vi "MainVI.vi"() -> ()   [LabVIEW 2013]
uses:
  Measurement.lvclass/Measurement.lvclass
  CSVExport.lvclass/CSVExport.lvclass
  SystemData.lvclass/SystemData.lvclass/SystemData.ctl
  Close.lvclass/Close.lvclass
  RootCommand.lvclass/RootCommand.lvclass
  Generator.lvclass/Generator.lvclass
  SystemData.lvclass/SystemData.lvclass
panel:
  in  "SignalGeneratorParameter":cluster{"Frequency":dbl, "Amplitude":dbl}={"Frequency"=10.0, "Amplitude"=1.0}
  in  "CSVExport":bool
  in  "Measurement":bool
  out "Waveform":waveform(dbl)(graph)
  in  "SourceSelect":u16(ring) items=["正弦波產生器", "方波產生器", "三角波產生器"]
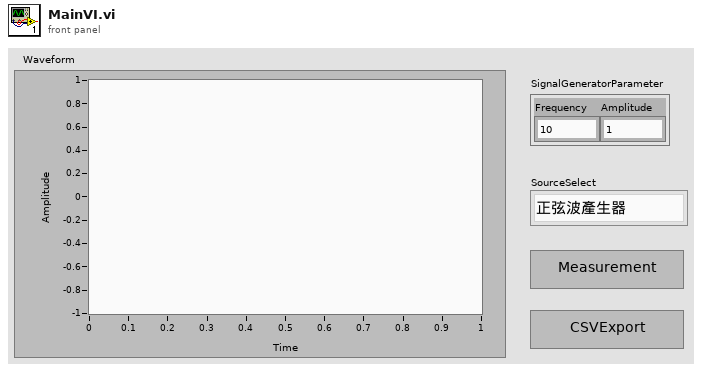
[diagram p1: front panel]
types:
  T1 = typedef "SystemData.lvclass/SystemDataTypeDefine.ctl" = cluster{"ThisVIParameter":cluster{"ThisVIPath":path, "ThisVIReference":refnum<vi>, "AllControlReference":refnum<vi>[]}, "GeneratorParameter":cluster{"Frequency":dbl, "Amplitude":dbl}, "WaveformBuffer":waveform(dbl), "SourceSelect":u16, "GeneratorClassArray":refnum<class "Generator.lvclass">[]}
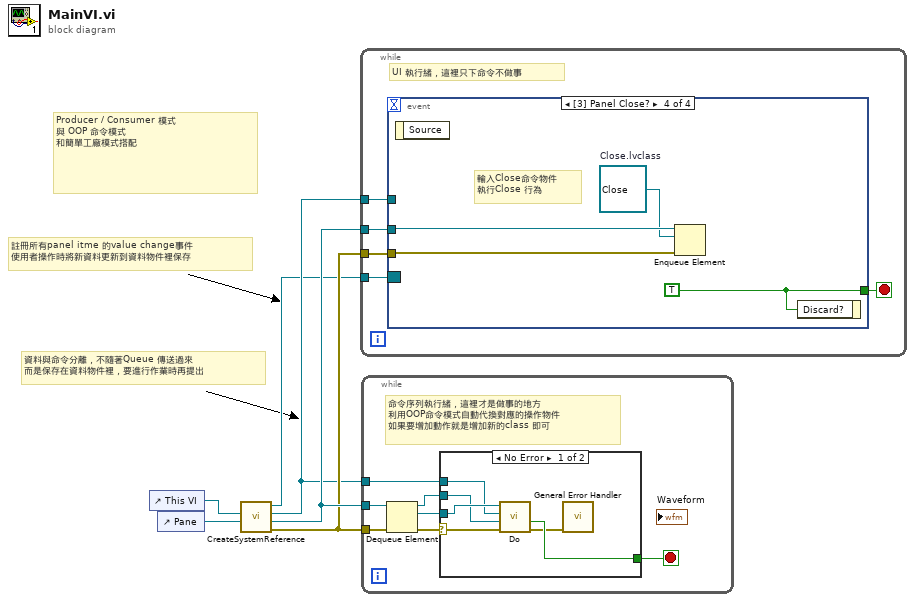
[diagram p0: block diagram]
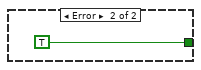
[diagram p2: hidden frame]
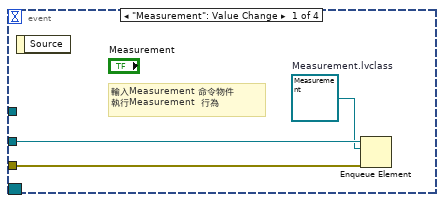
[diagram p3: hidden frame]
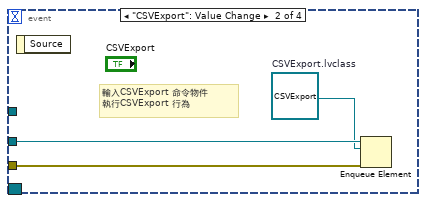
[diagram p4: hidden frame]
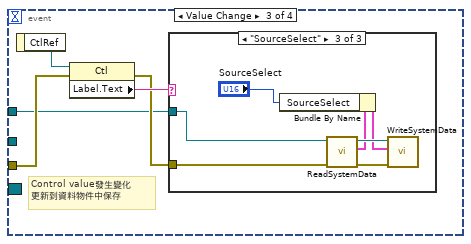
[diagram p5: hidden frame]
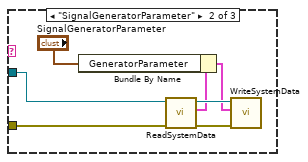
[diagram p7: hidden frame]
diagram:
  # "註冊所有panel itme 的value change事件\n使用者操作時將新資料更新到資料物件裡保存"
  # "資料與命令分離，不隨著Queue 傳送過來\n而是保存在資料物件裡，要進行作業時再提出"
  # "Producer / Consumer 模式\n與 OOP 命令模式\n和簡單工廠模式搭配"
  n1 = control-ref of="This VI"() -> (w5:refnum<vi>)
  n2 = control-ref of="Pane"() -> (w6:refnum<vi>)
  n3 = call "CreateSystemReference.vi"("Pane"=w6, "ThisVIReference"=w5) -> ("error out"=w3:errorcluster, "CommandQueueOut"=w4:refnum<queue>, "DataNotifierOut"=w2:refnum<notifier>, "ControlValueChangeEventRef"=w1:refnum<event-registration>)  [unwired: 6 in]
  n4 = while {
    tunnel: w4 -> [w11]
    tunnel: w3 -> [w10]
    tunnel: w2 -> [w9]
    tunnel: w1 -> [w8]
    stop <- w7 stop-if-true
    # "UI 執行緒，這裡只下命令不做事"
    n5 = event shown="[3] Panel Close?" {
      selector: w8 -> [_ _ _ _]
      dyn-events: _ -> [_ _ _ _]
      timeout: _ -> [_ _ _ _]
      tunnel: w11 -> [w14 w17 _ w38]
      tunnel: w10 -> [w13 w16 w21 w39]
      tunnel: [_ _ _ w40] -> w7
      tunnel: w9 -> [_ _ w18 _]
      event "Measurement": Value Change {
        w12 = refnum<class "Measurement.lvclass"> refnum  # Measurement.lvclass
        # "輸入Measurement 命令物件\n執行Measurement  行為"
        n6 = event-data() -> ()  [unwired: 1 in, 1 out]
        n7 = Enqueue Element(queue=w14, element=w12, error in (no error)=w13) -> ()  [unwired: 1 in, 3 out]
      }
      event "CSVExport": Value Change {
        w15 = refnum<class "CSVExport.lvclass"> refnum  # CSVExport.lvclass
        # "輸入CSVExport 命令物件\n執行CSVExport 行為"
        n8 = event-data() -> ()  [unwired: 1 in, 1 out]
        n9 = Enqueue Element(queue=w17, element=w15, error in (no error)=w16) -> ()  [unwired: 1 in, 3 out]
      }
      event Value Change {
        # "Control value發生變化\n更新到資料物件中保存"
        n10 = event-data() -> ("CtlRef"=w22:refnum<vi>)  [unwired: 1 in]
        n11 = property class="Ctl"(reference=w22, error in=w21) -> (error out=w19:errorcluster, "Label.Text"=w20:string)  [unwired: 1 out]
        n12 = case shown="\"SourceSelect\"" w20 {
          tunnel: w19 -> [_ w29 w36]
          tunnel: w18 -> [_ w26 w33]
          frame Default {
          }
          frame "SignalGeneratorParameter" {
            n13 = call "ReadSystemData.vi"("error in (no error)"=w29, "DataNotifierIn"=w26) -> ("error out"=w28:errorcluster, "SystemData"=w25:T1, "DataNotifierIn"=w27:refnum<notifier>)  [unwired: 7 in]
            n14 = Bundle By Name(cluster=w25, "GeneratorParameter"="SignalGeneratorParameter") -> (w24:T1)
            n15 = call "WriteSystemData.vi"("error in (no error)"=w28, "SystemData"=w24, "DataNotifierIn"=w27) -> ()  [unwired: 7 in, 2 out]
          }
          frame "SourceSelect" {
            n16 = call "ReadSystemData.vi"("error in (no error)"=w36, "DataNotifierIn"=w33) -> ("error out"=w35:errorcluster, "SystemData"=w32:T1, "DataNotifierIn"=w34:refnum<notifier>)  [unwired: 7 in]
            n17 = Bundle By Name(cluster=w32, "SourceSelect"="SourceSelect") -> (w31:T1)
            n18 = call "WriteSystemData.vi"("error in (no error)"=w35, "SystemData"=w31, "DataNotifierIn"=w34) -> ()  [unwired: 7 in, 2 out]
          }
        }
      }
      event Panel Close? {
        w37 = refnum<class "Close.lvclass"> refnum  # Close.lvclass
        w40 = TRUE ("Discard?")
        # "輸入Close命令物件\n執行Close 行為"
        n19 = event-data() -> ()  [unwired: 1 in, 1 out]
        n20 = Enqueue Element(queue=w38, element=w37, error in (no error)=w39) -> ()  [unwired: 1 in, 3 out]
        n21 = event-data("Discard?"=w40) -> ()  [unwired: 1 in, 1 out]
      }
    }
  }
  n22 = while {
    tunnel: w4 -> [w47]
    tunnel: w3 -> [w43]
    tunnel: w2 -> [w42]
    stop <- w44 stop-if-true
    # "命令序列執行緒，這裡才是做事的地方\n利用OOP命令模式自動代換對應的操作物件\n如果要增加動作就是增加新的class 即可"
    n23 = Dequeue Element(queue=w47, error in (no error)=w43) -> (queue out=w41:refnum<queue>, element=w45:refnum<class "RootCommand.lvclass">, error out=w46:errorcluster)  [unwired: 1 in, 1 out]
    n24 = case shown="No Error" w46 {
      selector: w46 -> [w53 _]
      tunnel: w45 -> [w52 _]
      tunnel: [w49 TRUE] -> w44
      tunnel: w42 -> [w51 _]
      tunnel: w41 -> [w50 _]
      frame No Error {
        n25 = call-dynamic "Do.vi"("error in (no error)"=w53, "CommandQueueIn"=w50, "DataNotifierIn"=w51, "RootCommand in"=w52) -> ("error out"=w48:errorcluster, "ExitFlag"=w49:bool)  [unwired: 4 in, 2 out]
        n26 = call <vilib>:"General Error Handler.vi"("error in (no error)"=w48) -> ()  [unwired: 10 in, 5 out]
      }
      frame Error {
      }
    }
  }
